vi "PRIME Telescope Convert HHMMSS to RA and DEC Angle.vi"(10 "Dec String":string, 11 "RA String":string) -> (1 "RA and DEC":T1, 2 "DEC":dbl, 3 "RA":dbl)   [LabVIEW 2021, in "PRIME Telescope.lvclass"]
uses:
  PRIME Telescope.lvclass
  typedefs/CC cluster RA and DEC.ctl
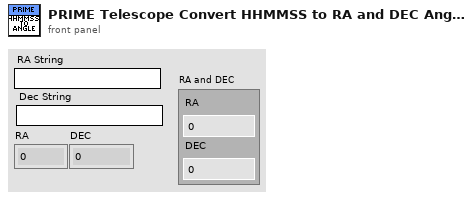
[diagram p1: front panel]
types:
  T1 = typedef "CC cluster RA and DEC.ctl" = cluster{"RA":dbl, "DEC":dbl}
  T2 = cluster{"hours":dbl, "Minutes":dbl, "seconds":dbl}
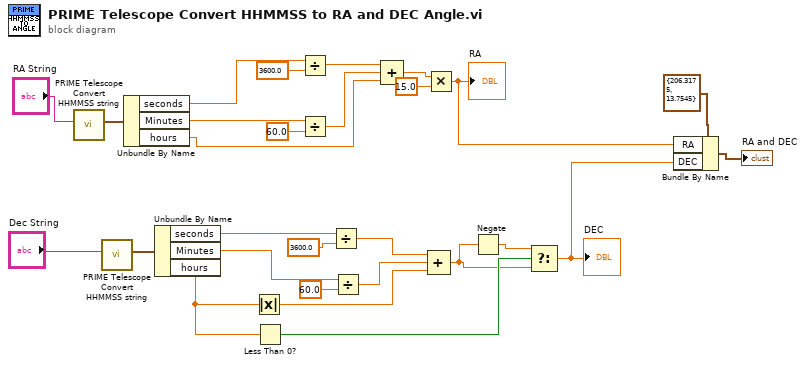
[diagram p0: block diagram]
diagram:
  n1 = call "PRIME Telescope Convert HHMMSS string.vi"("RA String"="RA String") -> ("Right Ascension"=w18:T2)  [unwired: 9 in, 1 out]
  n2 = call "PRIME Telescope Convert HHMMSS string.vi"("RA String"="Dec String") -> ("Right Ascension"=w14:T2)  [unwired: 9 in, 1 out]
  n3 = Unbundle By Name(w18) -> ("seconds"=w17:dbl, "Minutes"=w16:dbl, "hours"=w15:dbl)
  n4 = Unbundle By Name(w14) -> ("seconds"=w13:dbl, "Minutes"=w12:dbl, "hours"=w8:dbl)
  n5 = Absolute Value(x=w8) -> (abs(x)=w9:dbl)
  n6 = Less Than 0?(x=w8) -> (x < 0?=w7:bool)
  n7 = Divide(x=w17, y=3600.0) -> (x/y=w26:dbl)
  n8 = Divide(x=w16, y=60.0) -> (x/y=w25:dbl)
  n9 = Divide(x=w13, y=3600.0) -> (x/y=w11:dbl)
  n10 = Divide(x=w12, y=60.0) -> (x/y=w10:dbl)
  n11 = Compound Arithmetic op=ADD(w26, w25, w15) -> (w24:dbl)
  n12 = Multiply(x=w24, y=15.0) -> (x*y=w3:dbl)
  "RA" <- w3
  n13 = Compound Arithmetic op=ADD(w11, w10, w9) -> (w5:dbl)
  n14 = Negate(x=w5) -> (-x=w6:dbl)
  n15 = Select(t=w6, s=w7, f=w5) -> (s? t:f=w2:dbl)
  "DEC" <- w2
  n16 = Bundle By Name(cluster=T1 {"RA"=206.3175, "DEC"=13.7545} ("RA and DEC"), "RA"=w3, "DEC"=w2) -> (→"RA and DEC":T1)
